vi "GET ITEM INFO.vi"(11 "USER/ITEM DATA TRANSFER IN":T2(array[cluster])) -> (3 "ITEM DATA OUT":T1)   [LabVIEW 2019]
uses:
  Controls/Table Data Types/Inventory Data Type.ctl
  <vilib>/addons/database/Connection.llb/DB Tools Open Connec (String).vi
  <vilib>/addons/database/_DB Variant To Data/Database Variant To Data.xnode
  <vilib>/addons/database/NI_Database_API.lvlib
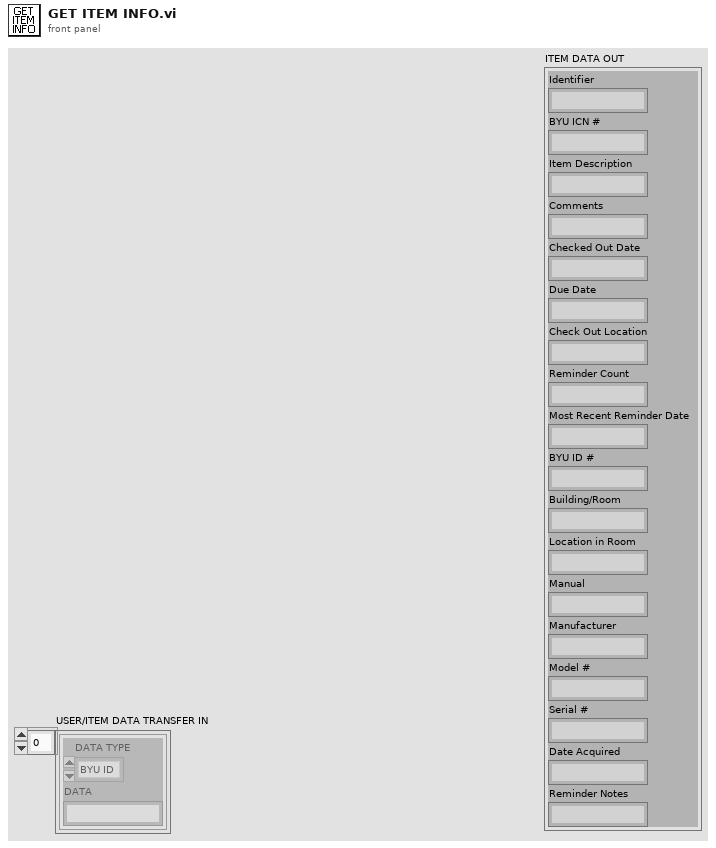
[diagram p1: front panel]
types:
  T1 = cluster{"Identifier":string, "BYU ICN #":string, "Item Description":string, "Comments":string, "Checked Out Date":string, "Due Date":string, "Check Out Location":string, "Reminder Count":string, "Most Recent Reminder Date":string, "BYU ID #":string, "Building/Room":string, "Location in Room":string, "Manual":string, "Manufacturer":string, "Model #":string, "Serial #":string, "Date Acquired":string, "Reminder Notes":string}
  T2 = cluster{"DATA TYPE":enum16{"BYU ID", "ME#/IDENTIFIER", "BYU ICN"}, "DATA":string}[]
  T3 = typedef "Inventory Data Type.ctl" = cluster{"Identifier":string, "BYU ICN #":string, "Item Description":string, "Comments":string, "Checked Out Date":string, "Due Date":string, "Check Out Location":string, "Reminder Count":i32, "Most Recent Reminder Date":string, "BYU ID #":string, "Building/Room":string, "Location in Room":string, "Manual":string, "Manufacturer":string, "Model #":string, "Serial #":string, "Date Acquired":string, "Reminder Notes":string}
  T4 = cluster{"DATA TYPE":enum16{"BYU ID", "ME#/IDENTIFIER", "BYU ICN"}, "DATA":string}
  T5 = typedef "NI_Database_API.lvlib/Conn ObjectReference.ctl" = refnum<k1>
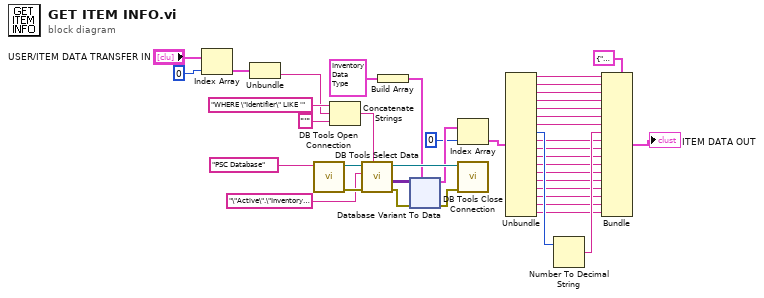
[diagram p0: block diagram]
diagram:
  n1 = Index Array(array="USER/ITEM DATA TRANSFER IN", index=0) -> (element=w40:T4)
  n2 = Unbundle(w40) -> ("DATA"=w34:string)  [unwired: 1 out]
  n3 = call-poly <vilib>:"DB Tools Open Connection.vi"("connection information"="PSC Database") -> ("error out"=w38:errorcluster, "connection reference"=w39:T5)  [unwired: 7 in]
  n4 = Concatenate Strings("WHERE \"Identifier\" LIKE '" ("string"), w34, "'" ("string")) -> (w33:string)
  n5 = call <vilib>:"DB Tools Select Data.vi"("condition"=w33, "error in (no error)"=w38, "table"="\"Active\".\"Inventory\"", "connection reference"=w39) -> ("error out"=w31:errorcluster, "data"=w30:variant[][], "connection reference out"=w28:T5)  [unwired: 2 in]
  n6 = Build Array(T3 {"Identifier"="", "BYU ICN #"="", "Item Description"="", "Comments"="", "Checked Out Date"="", "Due Date"="", "Check Out Location"="", "Reminder Count"=0, "Most Recent Reminder Date"="", "BYU ID #"="", "Building/Room"="", "Location in Room"="", "Manual"="", "Manufacturer"="", "Model #"="", "Serial #"="", "Date Acquired"="", "Reminder Notes"=""} ("INVENTORY DATA TYPE")) -> (w24:T3[])
  n7 = xnode "Database Variant To Data"("database variant"=w30, "error in (no error)"=w31, "type"=w24) -> ("data"=w27:T3[], "error out"=w29:errorcluster)
  n8 = Index Array(array=w27, index=0) -> (element=w23:T3)
  n9 = call <vilib>:"DB Tools Close Connection.vi"("error in (no error)"=w29, "connection reference"=w28) -> ()  [unwired: 5 in, 1 out]
  n10 = Unbundle(w23) -> ("Identifier"=w20:string, "BYU ICN #"=w19:string, "Item Description"=w18:string, "Comments"=w17:string, "Checked Out Date"=w16:string, "Due Date"=w15:string, "Check Out Location"=w14:string, "Reminder Count"=w13:i32, "Most Recent Reminder Date"=w11:string, "BYU ID #"=w10:string, "Building/Room"=w9:string, "Location in Room"=w8:string, "Manual"=w7:string, "Manufacturer"=w6:string, "Model #"=w5:string, "Serial #"=w4:string, "Date Acquired"=w3:string, "Reminder Notes"=w1:string)
  n11 = Number To Decimal String(number=w13) -> (decimal integer string=w12:string)  [unwired: 1 in]
  n12 = Bundle(cluster=T1 {"Identifier"="", "BYU ICN #"="", "Item Description"="", "Comments"="", "Checked Out Date"="", "Due Date"="", "Check Out Location"="", "Reminder Count"="", "Most Recent Reminder Date"="", "BYU ID #"="", "Building/Room"="", "Location in Room"="", "Manual"="", "Manufacturer"="", "Model #"="", "Serial #"="", "Date Acquired"="", "Reminder Notes"=""} ("ITEM DATA IN"), "Identifier"=w20, "BYU ICN #"=w19, "Item Description"=w18, "Comments"=w17, "Checked Out Date"=w16, "Due Date"=w15, "Check Out Location"=w14, "Reminder Count"=w12, "Most Recent Reminder Date"=w11, "BYU ID #"=w10, "Building/Room"=w9, "Location in Room"=w8, "Manual"=w7, "Manufacturer"=w6, "Model #"=w5, "Serial #"=w4, "Date Acquired"=w3, "Reminder Notes"=w1) -> (→"ITEM DATA OUT":T1)
